vi "hmi_halo_drive.vi"(4 "QuickTurn Const":dbl=0.15, 5 "Quickturn_Sens_Low":dbl=1.2, 7 "Speedturn_Sens_Low":dbl=1.0, 10 "Wheel":dbl, 11 "Throttle":dbl) -> (3 "Drive Data":cluster{"Left":dbl, "Right":dbl})   [LabVIEW 2014]
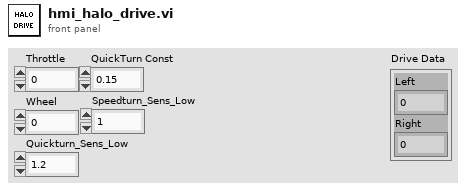
[diagram p1: front panel]
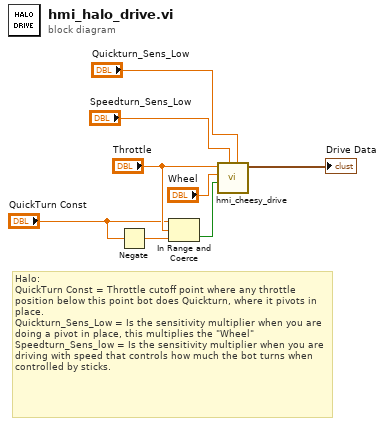
[diagram p0: block diagram]
diagram:
  # "Halo:\nQuickTurn Const = Throttle cutoff point where any throttle position below this point bot does Quickturn, where it pivots in place.\nQuickturn_Sens_Low = Is the sensitivity multiplier when you are doing a pivot in place, this multiplies the \"Wheel\" \nSpeedturn_Sens_low = Is the sensitivity multiplier when you are driving with speed that controls how much the bot turns when controlled by sticks."
  n1 = Negate(x="QuickTurn Const") -> (-x=w5:dbl)
  n2 = In Range and Coerce(upper limit="QuickTurn Const", x="Throttle", lower limit=w5) -> (In Range?=w3:bool)  [unwired: 1 out]
  n3 = call "hmi_cheesy_drive.vi"("Quickturn_Sens_Low"="Quickturn_Sens_Low", "Speedturn_Sens_Low"="Speedturn_Sens_Low", "Quick Turn"=w3, "Wheel"="Wheel", "Throttle"="Throttle") -> ("Drive Data"=→"Drive Data":cluster{"Left":dbl, "Right":dbl})  [unwired: 6 in]
